vi "Broken Arrow.vi"(8 "error in (no error)":errorcluster, 11 "Tamagotchi Full Actor in":refnum<class "Tamagotchi Full Actor.lvclass">) -> (0 "error out":errorcluster, 3 "Tamagotchi Full Actor out":refnum<class "Tamagotchi Full Actor.lvclass">)   [LabVIEW 2026, in "Tamagotchi Full Actor.lvclass"]
uses:
  Tamagotchi Full Actor.lvclass
  Tamagotchi Full Actor.lvclass/Tamagotchi Full Actor.ctl
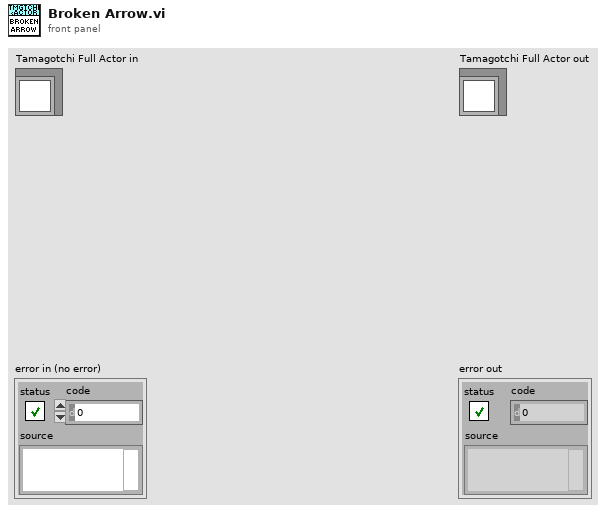
[diagram p1: front panel]
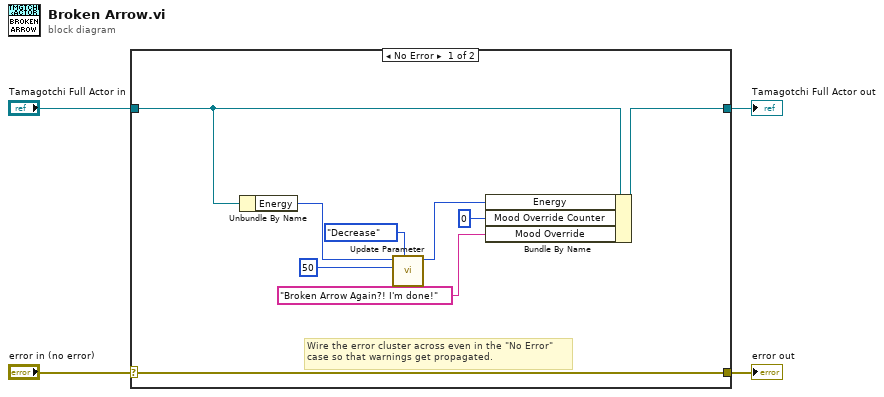
[diagram p0: block diagram]
diagram:
  n1 = case shown="No Error" "error in (no error)" {
    selector: "error in (no error)" -> [w13 w15]
    tunnel: [w13 w15] -> w3
    tunnel: [w6 w14] -> w1
    tunnel: "Tamagotchi Full Actor in" -> [w7 w14]
    frame No Error {
      # "Wire the error cluster across even in the \"No Error\"\ncase so that warnings get propagated."
      n2 = Unbundle By Name(w7) -> ("Energy"=w10:i16)
      n3 = call "Update Parameter.vi"("Action"=enum16{"Increase", "Decrease"}."Decrease", "Modifier"=i16 50 ("y"), "Parameter"=w10) -> ("New Value"=w11:i16)  [unwired: 8 in]
      n4 = Bundle By Name(cluster=w7, "Energy"=w11, "Mood Override Counter"=u32 0, "Mood Override"="Broken Arrow Again?! I'm done!") -> (w6:refnum<class "Tamagotchi Full Actor.lvclass">)
    }
    frame Error {
    }
  }
  "error out" <- w3
  "Tamagotchi Full Actor out" <- w1
